vi "Wait.vi"(8 "error in (no error)":errorcluster, 9 "Timeout (-1ms)":i32=-1, 11 "Response Core in":refnum<class "Interruptible Reply Core.lvclass">) -> (0 "error out":errorcluster, 1 "Timeout?":bool, 3 "Response Core out":refnum<class "Interruptible Reply Core.lvclass">)   [LabVIEW 2020, in "Publisher.lvlib" / "Interruptible Reply Core.lvclass"]
doc: "Execute a wait on the Response Core. \n\nThis implementation waits on the queue using the Preview method."
uses:
  Interruptible Reply Core.lvclass
  Interruptible Reply Core.lvclass/Interruptible Reply Core.ctl
  PPL/HDH.Data.Generic.lvlibp/Synchronization/Queue/Queue.lvclass
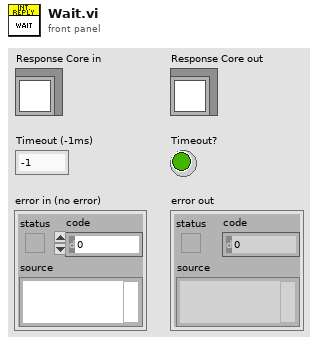
[diagram p1: front panel]
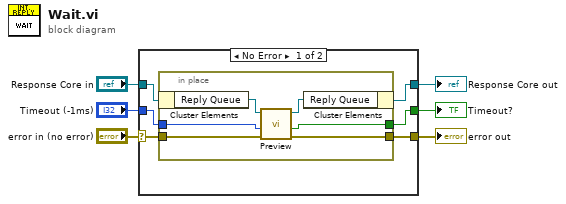
[diagram p0: block diagram]
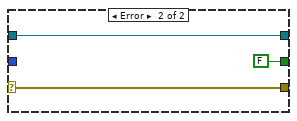
[diagram p2: hidden frame]
diagram:
  n1 = case shown="No Error" "error in (no error)" {
    selector: "error in (no error)" -> [w10 w21]
    tunnel: [w8 w21] -> w5
    tunnel: [w9 FALSE ("Dropped?")] -> w4
    tunnel: "Response Core in" -> [w12 w19]
    tunnel: [w7 w19] -> w2
    tunnel: "Timeout (-1ms)" -> [w11 _]
    frame No Error {
      n2 = in-place {
        in-place-border: w11 -> [w17]
        in-place-border: w10 -> [w16]
        in-place-border: [w15] -> w9
        in-place-border: [w14] -> w8
        n3 = in-place-cluster #1(w12) -> ("Reply Queue"=w18:refnum<class "Queue.lvclass">)
        n4 = call "Preview.vi"("error in (no error)"=w16, "timeout in ms (-1)"=w17, "Queue in"=w18) -> ("error out"=w14:errorcluster, "timed out?"=w15:bool, "Queue out"=w13:refnum<class "Queue.lvclass">)  [unwired: 5 in, 1 out]
        n5 = in-place-cluster #1("Reply Queue"=w13) -> (w7:refnum<class "Interruptible Reply Core.lvclass">)
      }
    }
    frame Error {
    }
  }
  "error out" <- w5
  "Response Core out" <- w2
  "Timeout?" <- w4
